vi "CalendarMouseover.vi"(8 "error in (no error)":errorcluster, 10 "Coords":T1, 11 "Calendar in":refnum<class "Calendar.lvclass">) -> (0 "error out":errorcluster, 3 "Calendar (dup)":refnum<class "Calendar.lvclass">)   [LabVIEW 2020, in "Calendar.lvclass"]
uses:
  Calendar.lvclass
  <vilib>/Utility/miscctls.llb/LVPoint32TypeDef.ctl
  Calendar.lvclass/Calendar.ctl
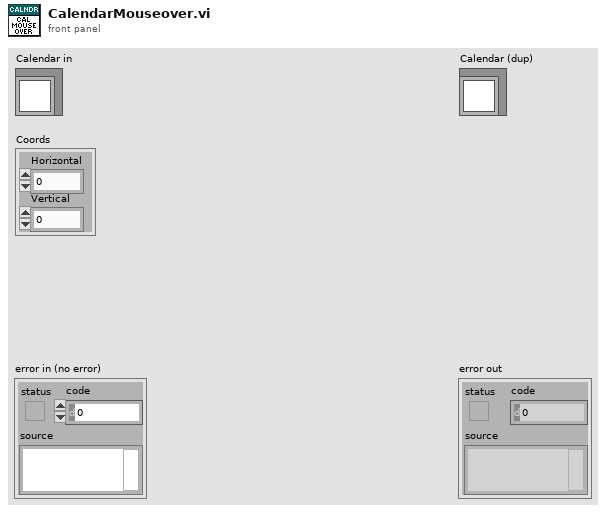
[diagram p1: front panel]
types:
  T1 = typedef "LVPoint32TypeDef.ctl" = cluster{"Horizontal":i32, "Vertical":i32}
  T2 = typedef "LVRowAndColumnTypeDef.ctl" = cluster{"Row":i32, "Column":i32}
  T3 = typedef "LVBoundsTypeDef.ctl" = cluster{"Width":u32, "Height":u32}
  T4 = typedef "LVPositionTypeDef.ctl" = cluster{"Left":i32, "Top":i32}
  T5 = typedef "LVPointTypeDef.ctl" = cluster{"Horizontal":i16, "Vertical":i16}
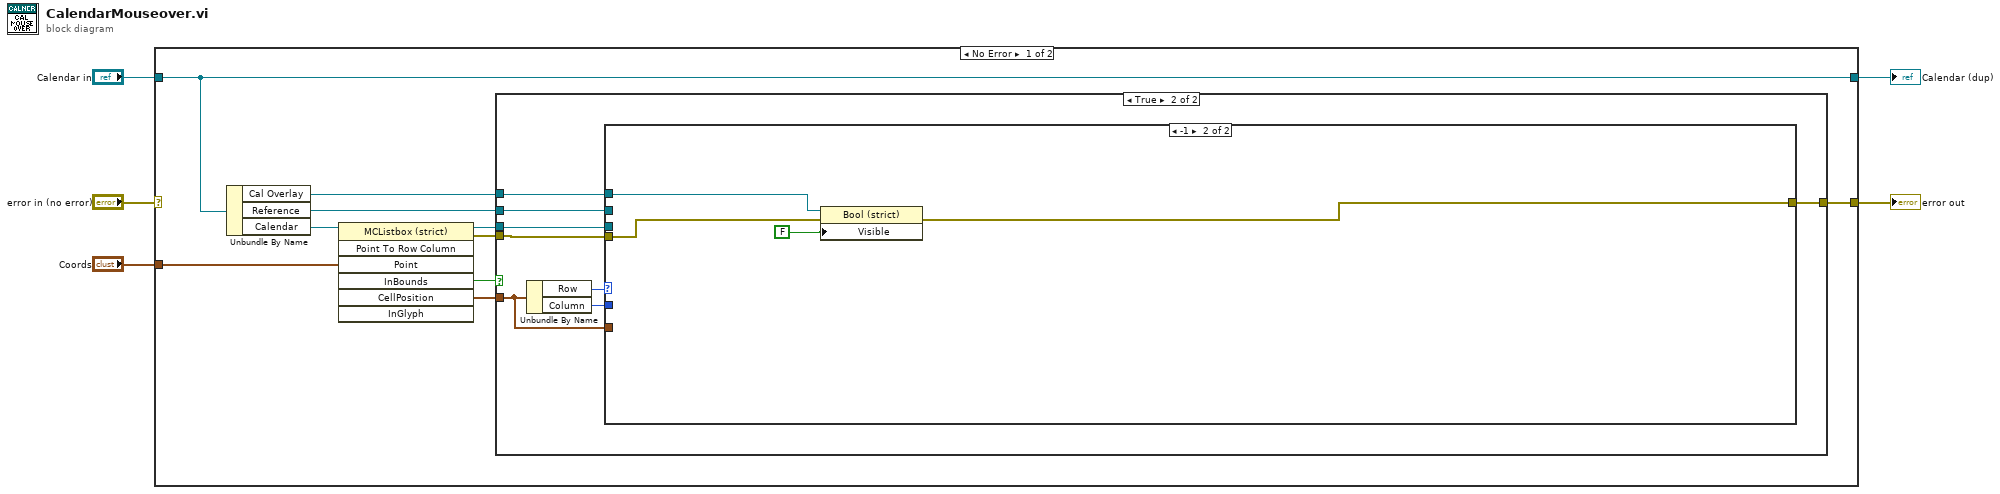
[diagram p0: block diagram]
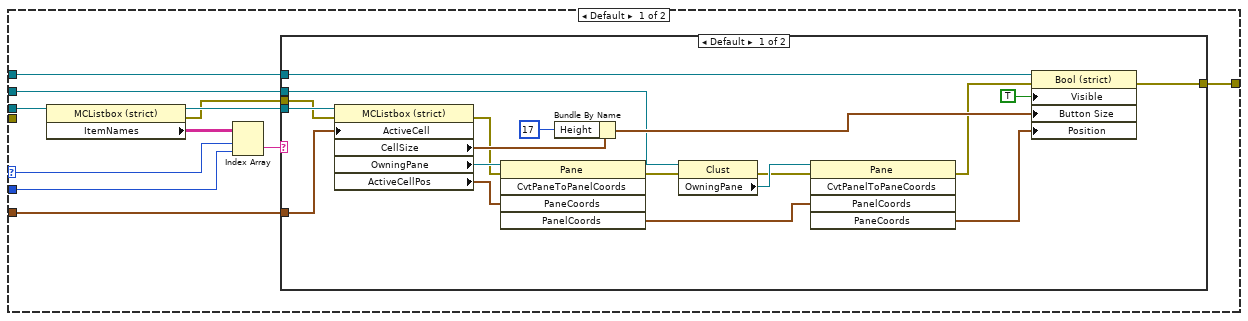
[diagram p3: hidden frame]
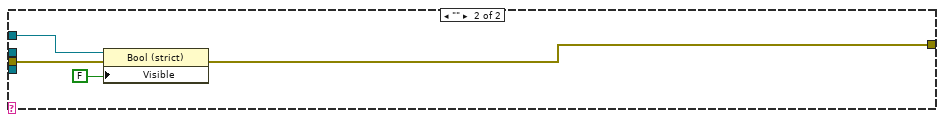
[diagram p4: hidden frame]
diagram:
  n1 = case shown="No Error" "error in (no error)" {
    selector: "error in (no error)" -> [_ w64]
    tunnel: [w8 w64] -> w4
    tunnel: [w15 w63] -> w2
    tunnel: "Calendar in" -> [w15 w63]
    tunnel: "Coords" -> [w13 _]
    frame No Error {
      n2 = Unbundle By Name(w15) -> ("Cal Overlay"=w6:refnum<vi>, "Reference"=w11:refnum<vi>, "Calendar"=w14:refnum<vi>)
      n3 = invoke class="MCListbox (strict)" method="Point To Row Column"(reference=w14, "Point"=w13) -> (reference out=w9:refnum<vi>, error out=w7:errorcluster, "InBounds"=w12:bool, "CellPosition"=w10:T2)  [unwired: 5 in, 3 out]
      n4 = case shown="True" w12 {
        tunnel: w11 -> [_ w23]
        tunnel: w10 -> [_ w20]
        tunnel: w9 -> [_ w22]
        tunnel: [w16 w19] -> w8
        tunnel: w7 -> [w16 w18]
        tunnel: w6 -> [_ w17]
        frame False {
        }
        frame True {
          n5 = Unbundle By Name(w20) -> ("Row"=w24:i32, "Column"=w21:i32)
          n6 = case shown="-1" w24 {
            selector: w24 -> [w33 _]
            tunnel: w23 -> [w30 _]
            tunnel: w22 -> [w35 _]
            tunnel: w21 -> [w32 _]
            tunnel: w20 -> [w28 _]
            tunnel: [w27 w61] -> w19
            tunnel: w18 -> [_ w60]
            tunnel: w17 -> [w25 w59]
            frame Default {
              n7 = property class="MCListbox (strict)"(reference=w35) -> (reference out=w29:refnum<vi>, error out=w26:errorcluster, "ItemNames"=w34:string[][])  [unwired: 1 in]
              n8 = Index Array(array=w34, index (row)=w33, index (col)=w32) -> (element=w31:string)
              n9 = case shown="Default" w31 {
                tunnel: w30 -> [w36 _]
                tunnel: w29 -> [w54 _]
                tunnel: w28 -> [w53 _]
                tunnel: [w52 w57] -> w27
                tunnel: w26 -> [w51 w56]
                tunnel: w25 -> [w37 w55]
                frame Default {
                  n10 = property on="Property Node" class="MCListbox (strict)"(reference=w54, error in=w51, "ActiveCell"=w53) -> (error out=w41:errorcluster, "CellSize"=w46:T3, "OwningPane"=w50:refnum<vi>, "ActiveCellPos"=w49:T4)  [unwired: 1 out]
                  n11 = invoke on="Invoke Node" class="Pane" method="CvtPaneToPanelCoords"(reference=w50, error in=w41, "PaneCoords"=w49) -> (error out=w40:errorcluster, "PanelCoords"=w43:T5)  [unwired: 2 in, 3 out]
                  n12 = Bundle By Name(cluster=w46, "Height"=u32 17) -> (w45:T3)
                  n13 = property class="Clust"(reference=w36, error in=w40) -> (error out=w39:errorcluster, "OwningPane"=w44:refnum<vi>)  [unwired: 1 out]
                  n14 = invoke on="Invoke Node" class="Pane" method="CvtPanelToPaneCoords"(reference=w44, error in=w39, "PanelCoords"=w43) -> (error out=w38:errorcluster, "PaneCoords"=w42:T5)  [unwired: 2 in, 3 out]
                  n15 = property class="Bool (strict)"(reference=w37, error in=w38, "Visible"=TRUE, "Button Size"=w45, "Position"=w42) -> (error out=w52:errorcluster)  [unwired: 1 out]
                }
                frame "" {
                  n16 = property class="Bool (strict)"(reference=w55, error in=w56, "Visible"=FALSE) -> (error out=w57:errorcluster)  [unwired: 1 out]
                }
              }
            }
            frame -1 {
              n17 = property class="Bool (strict)"(reference=w59, error in=w60, "Visible"=FALSE) -> (error out=w61:errorcluster)  [unwired: 1 out]
            }
          }
        }
      }
    }
    frame Error {
    }
  }
  "error out" <- w4
  "Calendar (dup)" <- w2
